vi "Set File Properties.vi"(7 "scope":T2, 8 "error in (no error)":errorcluster, 9 "properties":T1, 10 "owner":string, 11 "error list <top>":variant) -> (0 "error out":errorcluster, 3 "error list <top> out":variant)   [LabVIEW 2017]
uses:
  Scope.ctl
  Error Code File Properties.ctl
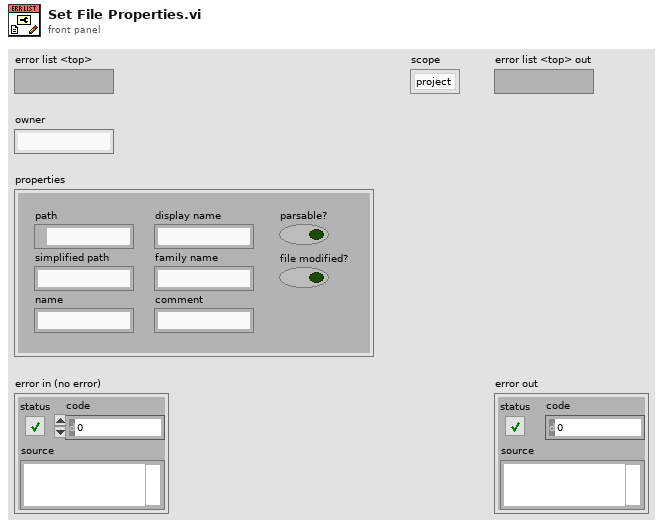
[diagram p1: front panel]
types:
  T1 = typedef "Error Code File Properties.ctl" = cluster{"path":path, "simplified path":string, "name":string, "display name":string, "family name":string, "comment":string, "parsable?":bool, "file modified?":bool}
  T2 = typedef "Scope.ctl" = enum16{"project", "global"}
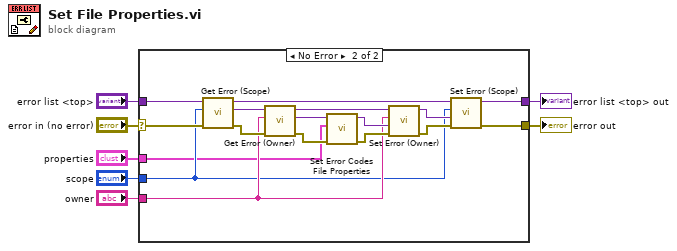
[diagram p0: block diagram]
diagram:
  n1 = case shown="No Error" "error in (no error)" {
    selector: "error in (no error)" -> [w9 w26]
    tunnel: "error list <top>" -> [w8 w15]
    tunnel: "owner" -> [_ w14]
    tunnel: "scope" -> [_ w11]
    tunnel: "properties" -> [_ w10]
    tunnel: [w9 w13] -> w2
    tunnel: [w8 w12] -> w1
    frame Error {
    }
    frame No Error {
      n2 = call "Get Error (Scope).vi"("error in (no error)"=w26, "scope"=w11, "error list <top>"=w15) -> ("error out"=w24:errorcluster, "error list <scope>"=w25:variant, "error list <top> dup"=w17:variant)  [unwired: 5 in, 1 out]
      n3 = call "Get Error (Owner).vi"("error in (no error)"=w24, "owner"=w14, "error list <scope>"=w25) -> ("error out"=w22:errorcluster, "error list <owner>"=w23:variant, "error list <scope> dup"=w20:variant)  [unwired: 5 in, 1 out]
      n4 = call "Set Error Codes File Properties.vi"("error in (no error)"=w22, "properties"=w10, "error list <owner> in"=w23) -> ("error out"=w19:errorcluster, "error list <owner> out"=w21:variant)  [unwired: 7 in]
      n5 = call "Set Error (Owner).vi"("error in (no error)"=w19, "error list <owner>"=w21, "owner"=w14, "error list <scope> in"=w20) -> ("error out"=w16:errorcluster, "error list <scope> out"=w18:variant)  [unwired: 6 in]
      n6 = call "Set Error (Scope).vi"("error in (no error)"=w16, "error list <scope>"=w18, "scope"=w11, "error list <top> in"=w17) -> ("error out"=w13:errorcluster, "error list <top> out"=w12:variant)  [unwired: 6 in]
    }
  }
  "error out" <- w2
  "error list <top> out" <- w1
